vi "19.1.-Data Socket de VIs con Código de LabVIEW (MASTER).vi"() -> ()   [LabVIEW 2020]
uses:
  <vilib>/measure/NI_MABase.lvlib
panel:
  out "error out":errorcluster
  out "Waveform Graph":waveform(dbl)(graph)
  in  "signal type":T1(ring)
  in  "phase":dbl(knob) scale=0.0..10.0
  in  "amplitude":dbl(knob)=1.0 scale=0.0..10.0
  in  "frequency":dbl(knob)=10.0 scale=0.0..10.0
  in  "URL":string
  in  "stop":bool
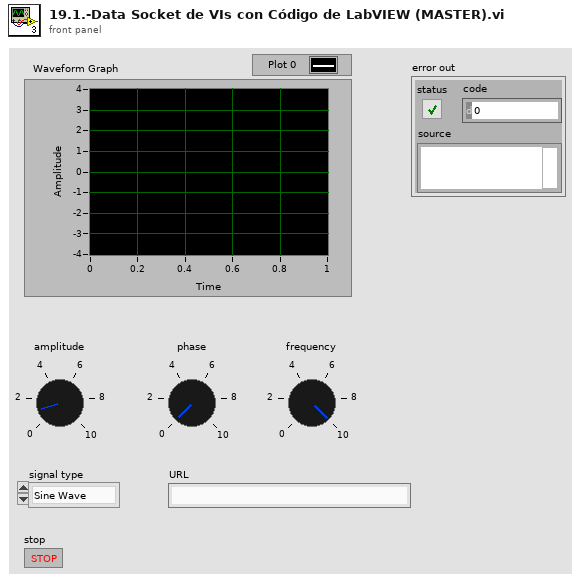
[diagram p1: front panel]
types:
  T1 = enum16{"Sine Wave", "Triangle Wave", "Square Wave", "Sawtooth Wave"}
  T2 = enum16{"Read", "Write", "ReadWrite", "BufferedRead", "BufferedReadWrite"}
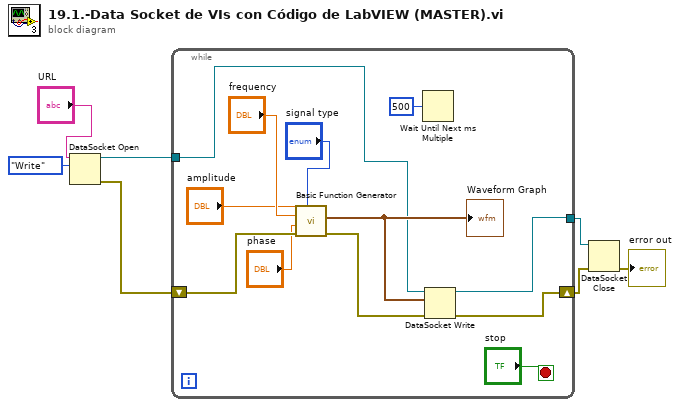
[diagram p0: block diagram]
diagram:
  n1 = DataSocket Open(10:T2."Write" ("mode"), 11:"URL") -> (0:w5:errorcluster, 3:w4:refnum<k13>)  [unwired: 2 in]
  n2 = while {
    shift-right: [w10] -> w2
    shift-left: w5 -> [w18]
    tunnel: w4 -> [w9]
    tunnel: [w8] -> w3
    stop <- "stop" stop-if-true
    n3 = call <vilib>:"Basic Function Generator.vi"("signal type"="signal type", "error in (no error)"=w18, "phase"="phase", "amplitude"="amplitude", "frequency"="frequency") -> ("error out"=w12:errorcluster, "signal out"=w11:waveform(dbl))  [unwired: 4 in, 1 out]
    "Waveform Graph" <- w11
    n4 = Wait Until Next ms Multiple(millisecond multiple=u32 500) -> ()  [unwired: 1 out]
    n5 = DataSocket Write(8:w12, 10:w11, 11:w9) -> (0:w10:errorcluster, 3:w8:refnum<k13>)  [unwired: 1 in, 1 out]
  }
  n6 = DataSocket Close(8:w2, 11:w3) -> (0:→"error out":errorcluster)  [unwired: 1 in, 1 out]
